vi "Create Statement from SQL.vi"(8 "error in (no error)":errorcluster, 9 "Num records":i32, 10 "SQL Dataset":variant[][](array[variant]), 11 "First Importing Credit Record":refnum<class "Credit Record.lvclass">) -> (0 "error out":errorcluster, 3 "Overlapping Recods":refnum<class "Statement.lvclass">)   [LabVIEW 2018, in "Credit Record.lvclass"]
uses:
  Credit Record.lvclass
  C:/Users/jtipps/Documents/Filthy-Lucre-Budgetizer/source/support/classes/Transaction/Transaction.lvclass
  Statement/Statement.lvclass
  Credit Statement/Credit Statement.lvclass
  C:/Users/jtipps/Documents/Filthy-Lucre-Budgetizer/source/support/classes/Statement/Statement.lvclass
  Statement/Statement.lvclass/Statement.ctl
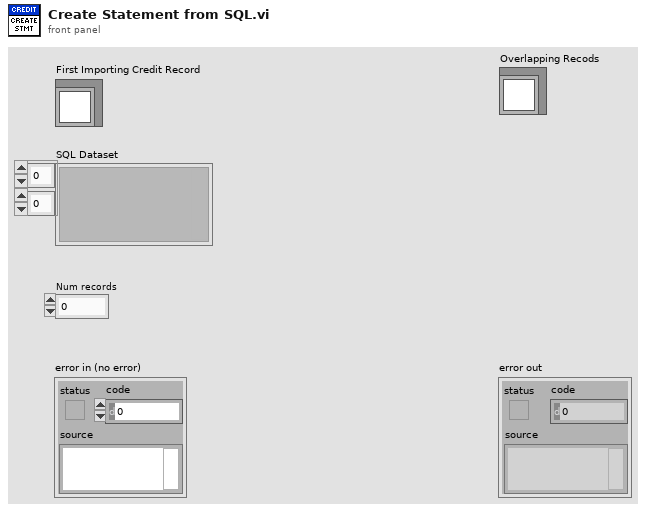
[diagram p1: front panel]
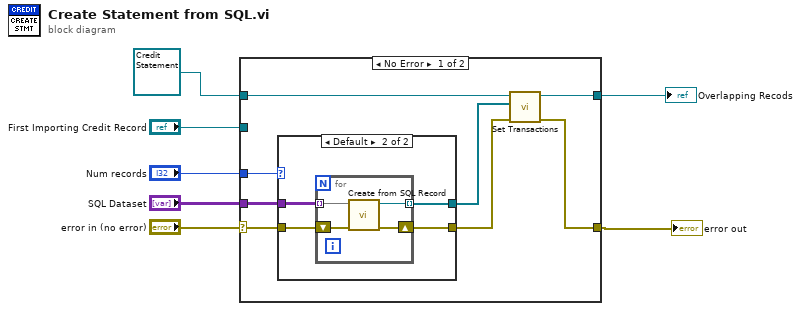
[diagram p0: block diagram]
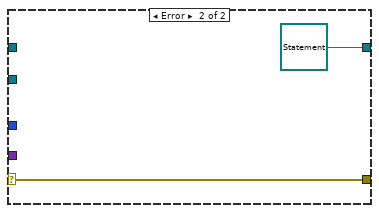
[diagram p3: hidden frame]
diagram:
  n1 = case shown="No Error" "error in (no error)" {
    selector: "error in (no error)" -> [w15 w26]
    tunnel: "Num records" -> [w14 _]
    tunnel: refnum<class "Credit Statement.lvclass"> refnum ("Credit Statement.lvclass") -> [w12 _]
    tunnel: "SQL Dataset" -> [w13 _]
    tunnel: [w8 w26] -> w3
    tunnel: [w11 refnum<class "Statement.lvclass"> refnum ("Statement out")] -> w1
    tunnel: "First Importing Credit Record" -> [_ _]
    frame No Error {
      n2 = case shown="Default" w14 {
        tunnel: w15 -> [w16 w20]
        tunnel: [w16 w19] -> w9
        tunnel: w13 -> [_ w18]
        tunnel: [_ w17] -> w10
        frame 0 {
        }
        frame Default {
          n3 = for {
            shift-right: [w21] -> w19
            shift-left: w20 -> [w22]
            tunnel: w18 -> [w24] mode=indexing
            tunnel: [w23] -> w17 mode=indexing
            n4 = call "Create from SQL Record.vi"("error in (no error)"=w22, "MySQL Record"=w24) -> ("error out"=w21:errorcluster, "Credit Record out"=w23:refnum<class "Credit Record.lvclass">)  [unwired: 8 in]
          }
        }
      }
      n5 = call "Set Transactions.vi"("error in (no error)"=w9, "Transactions"=w10, "Statement in"=w12) -> ("error out"=w8:errorcluster, "Statement out"=w11:refnum<class "Credit Statement.lvclass">)  [unwired: 7 in]
    }
    frame Error {
    }
  }
  "error out" <- w3
  "Overlapping Recods" <- w1
